vi "Demo-Browse.vi"() -> ()   [LabVIEW 2017]
uses:
  opcua-lvlib/Browser/Server Classes/UA Server/UA Server.lvclass
  opcua-lvlib/Server/Server.lvclass
  opcua-lvlib/TypeDefs/Data Type.ctl
  opcua-lvlib/opcua.lvlib
  opcua-lvlib/Client/Client.lvclass
  opcua-lvlib/Browser/Server Classes/Base Tree/Base Tree.lvclass
panel:
  out "# Nodes":i32
  in  "Tree":string(tree)
  out "MyVariable (Client)":i32
  out "My Variable (Server)":i32
  in  "Stop Button":bool
  # "Warning!  Please use the Stop Button at all times and not Abort Execution by LabVIEW. \nOtherwise, the handles will not be closed, and you will get an Exception next time. \nThis is because Process Detach/Thread Detach are not handled yet. Gets changed later."
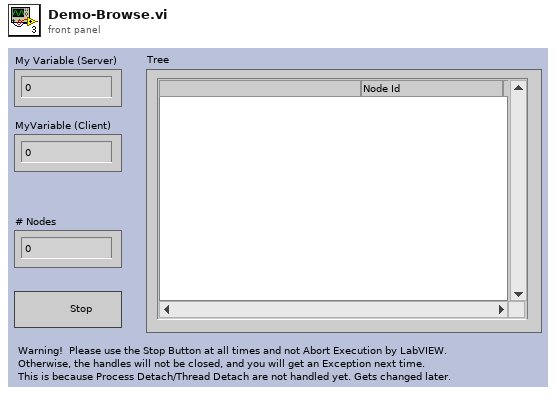
[diagram p1: front panel]
types:
  T1 = typedef "opcua.lvlib/Data Type.ctl" = u16
  T2 = enum32{"invalid app kind", "Development System", "Run Time System", "Student Edition", "Embedded LabVIEW", "Evaluation", "Custom"}
  T3 = typedef "opcua.lvlib/Node.ctl" = cluster{"class":i32, "Display Name":string, "Node UID":string}
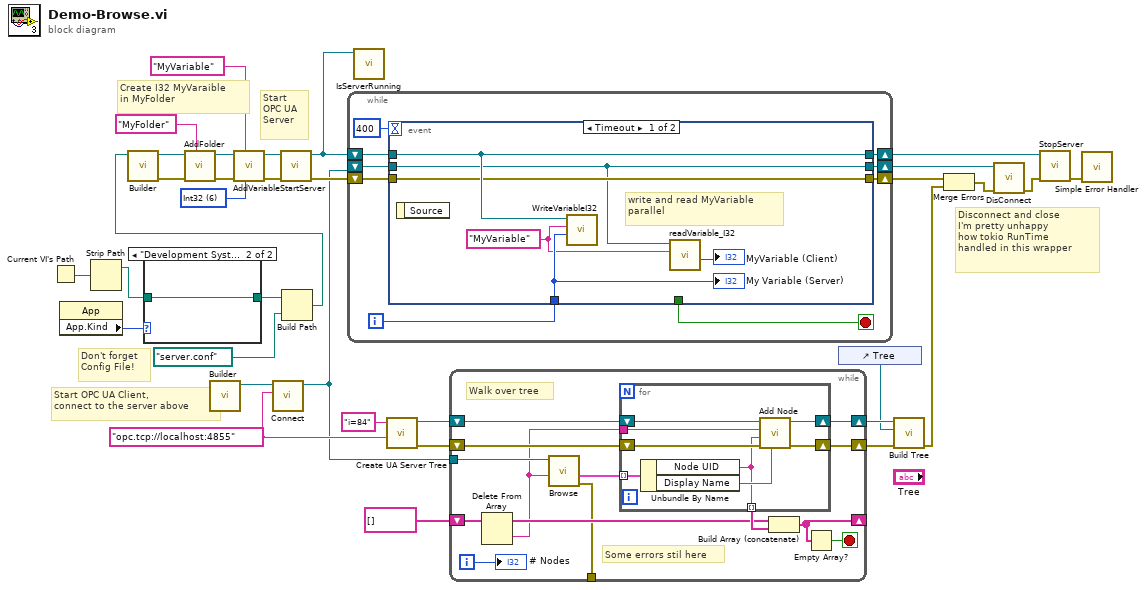
[diagram p0: block diagram]
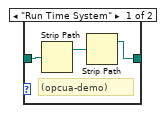
[diagram p2: hidden frame]
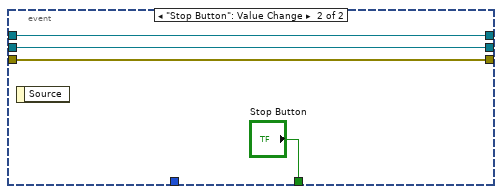
[diagram p3: hidden frame]
diagram:
  w15 = "opc.tcp://localhost:4855" ("URL")
  w27 = T1 6 items=["Boolean"=1, "SByte"=2, "Byte"=3, "Int16"=4, "UInt16"=5, "Int32"=6, "UInt32"=7, "Int64"=8, "UInt64"=9, "Float"=10, "Double"=11, "String"=12, "DateTime"=13, "ByteString"=15, "Array of Boolean"=101, "Array of SByte"=102, "Array of Byte"=103, "Array of Int16"=104, "Array of UInt16"=105, "Array of Int32"=106, "Array of UInt32"=107, "Array of Int64"=108, "Array of UInt64"=109, "Array of Float"=110, "Array of Double"=111, "Array of String"=112, "Array of DateTime"=113, "Array of ByteString"=115, "Matrix of Boolean"=201, "Matrix of SByte"=202, "Matrix of Byte"=203, "Matrix of Int16"=204, "Matrix of UInt16"=205, "Matrix of Int32"=206, "Matrix of UInt32"=207, "Matrix of Int64"=208, "Matrix of UInt64"=209, "Matrix of Float"=210, "Matrix of Double"=211, "Matrix of String "=212, "Matrix of DateTime"=213, "Matrix of ByteString"=215] ("type")
  # "Create I32 MyVaraible\nin MyFolder"
  # "Disconnect and close\nI'm pretty unhappy\nhow tokio RunTime\nhandled in this wrapper"
  # "Start OPC UA Client,\nconnect to the server above"
  # "Don't forget\nConfig File!"
  # "Start\nOPC UA\nServer"
  n1 = Current VI's Path() -> (path=w30:path)
  n2 = property class="App"() -> ("App.Kind"=w4:T2)  [unwired: 2 in, 2 out]
  n3 = Strip Path(path=w30) -> (stripped path=w3:path)  [unwired: 1 out]
  n4 = case shown="\"Development System\", Default" w4 {
    tunnel: w3 -> [w37 w38]
    tunnel: [w35 w38] -> w2
    frame "Run Time System" {
      # "(opcua-demo)"
      n5 = Strip Path(path=w37) -> (stripped path=w36:path)  [unwired: 1 out]
      n6 = Strip Path(path=w36) -> (stripped path=w35:path)  [unwired: 1 out]
    }
    frame "Development System", Default {
    }
  }
  n7 = call "Builder.vi"() -> ("Client out"=w16:refnum<class "Client.lvclass">)  [unwired: 10 in, 1 out]
  n8 = call "Connect.vi"("URL"=w15, "Client In"=w16) -> ("Client out"=w7:refnum<class "Client.lvclass">)  [unwired: 7 in, 2 out]
  n9 = Build Path(base path=w2, name or relative path=path "server.conf" ("Config File Path")) -> (appended path=w1:path)
  n10 = call "Builder.vi"("Config File Path"=w1) -> ("error out"=w33:errorcluster, "Server out"=w34:refnum<class "Server.lvclass">)  [unwired: 8 in, 1 out]
  n11 = call-dynamic "AddFolder.vi"("folder_node"="MyFolder", "error in (no error)"=w33, "Server in"=w34) -> ("error out"=w25:errorcluster, "Server out"=w26:refnum<class "Server.lvclass">)  [unwired: 7 in]
  n12 = call-dynamic "AddVariable.vi"("type"=w27, "variable_node"="MyVariable" ("folder_node"), "error in (no error)"=w25, "Server in"=w26) -> ("error out"=w31:errorcluster, "Server out"=w24:refnum<class "Server.lvclass">)  [unwired: 6 in]
  n13 = call-dynamic "StartServer.vi"("error in (no error)"=w31, "Server in"=w24) -> ("error out"=w20:errorcluster, "Server out"=w22:refnum<class "Server.lvclass">)  [unwired: 8 in]
  n14 = while {
    shift-right: [w43] -> w23
    shift-left: w22 -> [w46]
    shift-right: [w42] -> w19
    shift-left: w20 -> [w41]
    shift-right: [w40] -> w6
    shift-left: w7 -> [w39]
    i -> [w45]
    stop <- w44 stop-if-true
    n15 = event shown="[0] Timeout" {
      selector: _ -> [_ _]
      dyn-events: _ -> [_ _]
      timeout: 400 -> [_ _]
      tunnel: w46 -> [w53 w56]
      tunnel: w45 -> [w50 _]
      tunnel: [_ "Stop Button"] -> w44
      tunnel: [w53 w56] -> w43
      tunnel: [w52 w55] -> w42
      tunnel: w41 -> [w52 w55]
      tunnel: [w49 w54] -> w40
      tunnel: w39 -> [w49 w54]
      event Timeout {
        w48 = "MyVariable" ("folder_node")
        # "write and read MyVariable\nparallel"
        n16 = event-data() -> ()  [unwired: 1 in, 1 out]
        n17 = call-dynamic "WriteVariableI32.vi"("value"=w50, "variable_node"=w48, "Server in"=w53) -> ()  [unwired: 7 in, 2 out]
        n18 = call "readVariable_I32.vi"("URL"=w48, "Client In"=w49) -> ("val"=→"MyVariable (Client)":i32)  [unwired: 6 in, 3 out]
        "My Variable (Server)" <- w50
      }
      event "Stop Button": Value Change {
        n19 = event-data() -> ()  [unwired: 1 in, 1 out]
      }
    }
  }
  n20 = call-dynamic "IsServerRunning.vi"("Server in"=w22) -> ()  [unwired: 8 in, 3 out]
  n21 = call "Create UA Server Tree.vi"("Display Name"=w15, "Server Endpoint URL (Root folder)"="i=84" ("Display Name")) -> ("Error Out"=w10:errorcluster, "UA Server Tree"=w11:refnum<class "UA Server.lvclass">)  [unwired: 8 in]
  n22 = while {
    shift-right: [w67] -> w14
    shift-left: w11 -> [w71]
    shift-right: [w69] -> _
    shift-left: string[] [] -> [w66]
    tunnel: w7 -> [w62]
    shift-right: [w63] -> w12
    shift-left: w10 -> [w64]
    tunnel: [w59] -> _
    i -> [w60]
    stop <- w68 stop-if-true
    # "Some errors stil here"
    # "Walk over tree"
    n23 = Delete From Array(array=w66) -> (deleted portion=w58:string, array with subset deleted=w65:string[])  [unwired: 2 in]
    n24 = call "Browse.vi"("id as String"=w58, "Client In"=w62) -> ("error out"=w59:errorcluster, "result"=w61:T3[])  [unwired: 6 in, 2 out]
    n25 = for {
      tunnel: w61 -> [w78] mode=indexing
      tunnel: w58 -> [w73]
      tunnel: [w72] -> w70 mode=indexing
      shift-right: [w77] -> w67
      shift-left: w71 -> [w79]
      shift-right: [w75] -> w63
      shift-left: w64 -> [w76]
      n26 = Unbundle By Name(w78) -> ("Node UID"=w72:string, "Display Name"=w74:string)
      n27 = call-dynamic "Add Node.vi"("Display Name"=w74, "error in (no error)"=w76, "UID"=w72, "Parent"=w73, "Base Tree in"=w79) -> ("error out"=w75:errorcluster, "Base Tree out"=w77:refnum<class "UA Server.lvclass">)  [unwired: 5 in]
    }
    n28 = Build Array (concatenate)(w65, w70) -> (w69:string[])
    n29 = Empty Array?(array=w69) -> (empty?=w68:bool)
    "# Nodes" <- w60
  }
  n30 = control-ref of="Tree"() -> (w9:refnum<vi>)
  n31 = call "Build Tree.vi"("error in (no error)"=w12, "Tree Reference"=w9, "Base Tree in"=w14) -> ("error out"=w5:errorcluster)  [unwired: 7 in, 1 out]
  n32 = Merge Errors(w19, w5) -> (w18:errorcluster)
  n33 = call "DisConnect.vi"("error in (no error)"=w18, "Client In"=w6) -> ("error out"=w21:errorcluster)  [unwired: 7 in, 2 out]
  n34 = call-dynamic "StopServer.vi"("error in (no error)"=w21, "Server in"=w23) -> ("error out"=w17:errorcluster)  [unwired: 7 in, 2 out]
  n35 = call <vilib>:"Simple Error Handler.vi"("error in (no error)"=w17) -> ()  [unwired: 4 in, 5 out]
